vi "Monitor Data Changed.vi"(8 "error in (no error)":errorcluster, 9 "Changed Actor's Q":refnum<class "Message Enqueuer.lvclass">, 10 "Monitor Data":refnum<class "Monitor Data.lvclass">, 11 "Special Monitor New in":refnum<class "Special Monitor.lvclass">) -> (0 "error out":errorcluster, 3 "Special Monitor New out":refnum<class "Special Monitor.lvclass">)   [LabVIEW 2020, in "Special Monitor.lvclass"]
doc: "Called any time the monitor data is changed. Use the \"Changed Actor's Q\" to determine what actor has changed.\n\nCopyright: MGI 2016\nAuthor: Derek Trepanier"
uses:
  Special Monitor.lvclass
  <vilib>/MGI/Monitored Actor/Monitor Data/Monitor Data.lvclass
  <vilib>/ActorFramework/Message Enqueuer/Message Enqueuer.lvclass
  Special Monitor.lvclass/Special Monitor.ctl
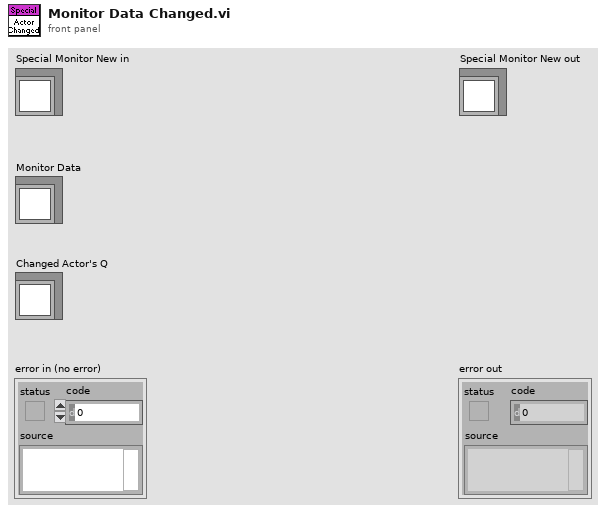
[diagram p1: front panel]
types:
  T1 = cluster{"Monitor Data":refnum<class "Monitor Data.lvclass">, "Changed Actor's Q":refnum<class "Message Enqueuer.lvclass">}
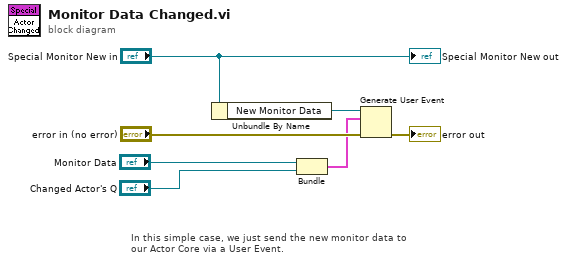
[diagram p0: block diagram]
diagram:
  # "In this simple case, we just send the new monitor data to\nour Actor Core via a User Event."
  n1 = Unbundle By Name("Special Monitor New in") -> ("New Monitor Data"=w4:refnum<user-event>)
  n2 = Bundle("Monitor Data"="Monitor Data", "Changed Actor's Q"="Changed Actor's Q") -> (w1:T1)  [unwired: 1 in]
  n3 = Generate User Event(user event=w4, event data cluster=w1, error in="error in (no error)") -> (error out=→"error out":errorcluster)  [unwired: 1 in, 1 out]
  "Special Monitor New out" <- "Special Monitor New in"
